vi "Close Reference.vi"(8 "error in (no error)":errorcluster, 11 "Listener In.lvclass":refnum<class "Listener.lvclass">) -> (0 "error out":errorcluster, 3 "Listener out":refnum<class "Listener.lvclass">)   [LabVIEW 2019, in "Listener.lvclass"]
uses:
  Listener.lvclass
  Listener.lvclass/Listener.ctl
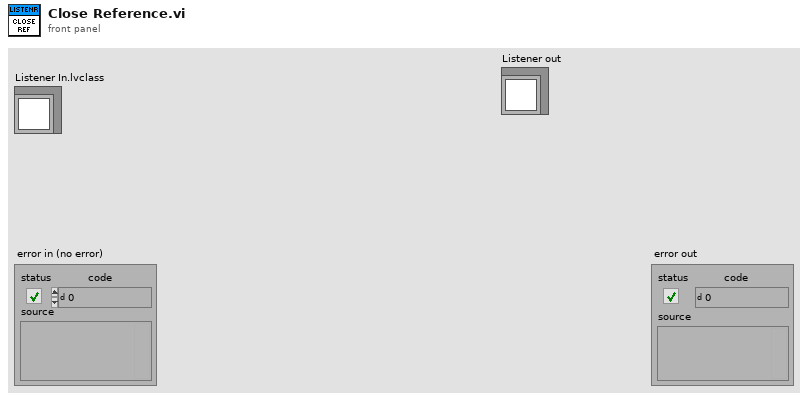
[diagram p1: front panel]
types:
  T1 = typedef "Listener.lvclass/Protocol.ctl" = enum16{"RS-XXX", "AK RS-XXX", "VISA", "TCPIP", "AK TCPIP", "UDP", "GPIB ConvBox"}
  T2 = typedef "Listener.lvclass/TCP Data Structure.ctl" = cluster{"TCP|IP connection ID":refnum<k5>, "IP Address":string, "Port":u16, "Data":string}
  T3 = typedef "Listener.lvclass/UDP Data Structure.ctl" = cluster{"UDP connection ID":refnum<k16>, "Local Address":string, "Local Port":u16, "Target IP Address":string, "Target Port":u16, "Data":string}
  T4 = typedef "Listener.lvclass/AK TCP Data Structure.ctl" = cluster{"TCP|IP connection ID":refnum<k5>, "IP Address":string, "Port":u16, "Data":string, "Current Command Code":string}
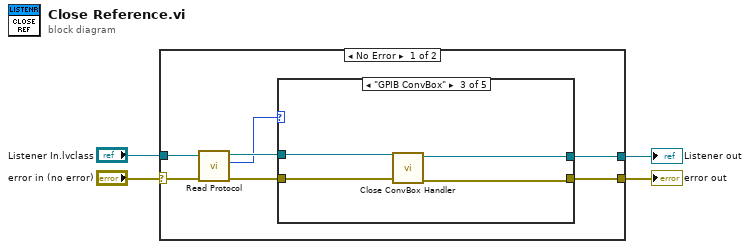
[diagram p0: block diagram]
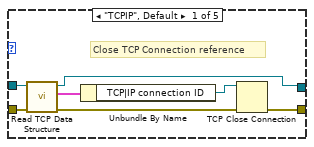
[diagram p2: hidden frame]
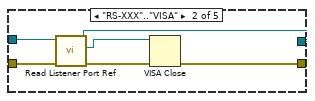
[diagram p3: hidden frame]
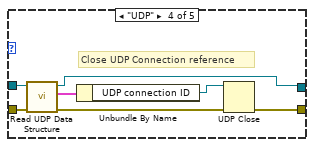
[diagram p4: hidden frame]
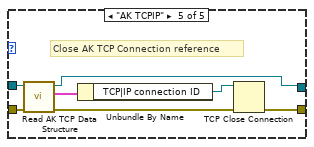
[diagram p5: hidden frame]
diagram:
  n1 = case shown="No Error" "error in (no error)" {
    selector: "error in (no error)" -> [w9 w44]
    tunnel: [w7 w44] -> w3
    tunnel: "Listener In.lvclass" -> [w11 w43]
    tunnel: [w6 w43] -> w1
    frame No Error {
      n2 = call-dynamic "Read Protocol.vi"("error in (no error)"=w9, "Listener in"=w11) -> ("error out"=w8:errorcluster, "Protocol"=w5:T1, "Listener out"=w10:refnum<class "Listener.lvclass">)  [unwired: 7 in]
      n3 = case shown="\"GPIB ConvBox\"" w5 {
        tunnel: w10 -> [w17 w21 w27 w35 w38]
        tunnel: w8 -> [w18 w23 w28 w34 w40]
        tunnel: [w14 w24 w26 w30 w41] -> w7
        tunnel: [w12 w19 w25 w29 w36] -> w6
        frame "TCPIP", Default {
          # "Close TCP Connection reference"
          n4 = call-dynamic "Read TCP Data Structure.vi"("error in (no error)"=w18, "Listener in"=w17) -> ("error out"=w15:errorcluster, "TCP|IP Data Structure"=w16:T2, "Listener out"=w12:refnum<class "Listener.lvclass">)  [unwired: 7 in]
          n5 = Unbundle By Name(w16) -> ("TCP|IP connection ID"=w13:refnum<k5>)
          n6 = TCP Close Connection(connection ID=w13, error in (no error)=w15) -> (error out=w14:errorcluster)  [unwired: 1 in, 1 out]
        }
        frame "RS-XXX".."VISA" {
          n7 = call "Read Listener Port Ref.vi"("error in (no error)"=w23, "Listener in"=w21) -> ("error out"=w22:errorcluster, "Listener Port Ref"=w20:refnum<visa-resource-name>, "Listener out"=w19:refnum<class "Listener.lvclass">)  [unwired: 7 in]
          n8 = VISA Close(VISA resource name=w20, error in (no error)=w22) -> (error out=w24:errorcluster)
        }
        frame "GPIB ConvBox" {
          n9 = call "Close ConvBox Handler.vi"("error in (no error)"=w28, "Listener in"=w27) -> ("error out"=w26:errorcluster, "Listener out"=w25:refnum<class "Listener.lvclass">)  [unwired: 8 in]
        }
        frame "UDP" {
          # "Close UDP Connection reference"
          n10 = call-dynamic "Read UDP Data Structure.vi"("error in (no error)"=w34, "Listener in"=w35) -> ("error out"=w32:errorcluster, "UDP Data Structure"=w33:T3, "Listener out"=w29:refnum<class "Listener.lvclass">)  [unwired: 7 in]
          n11 = Unbundle By Name(w33) -> ("UDP connection ID"=w31:refnum<k16>)
          n12 = UDP Close(connection ID=w31, 8:w32) -> (error out=w30:errorcluster)  [unwired: 1 out]
        }
        frame "AK TCPIP" {
          # "Close AK TCP Connection reference"
          n13 = call-dynamic "Read AK TCP Data Structure.vi"("error in (no error)"=w40, "Listener in"=w38) -> ("error out"=w39:errorcluster, "TCP|IP Data Structure"=w37:T4, "Listener out"=w36:refnum<class "Listener.lvclass">)  [unwired: 7 in]
          n14 = Unbundle By Name(w37) -> ("TCP|IP connection ID"=w42:refnum<k5>)
          n15 = TCP Close Connection(connection ID=w42, error in (no error)=w39) -> (error out=w41:errorcluster)  [unwired: 1 in, 1 out]
        }
      }
    }
    frame Error {
    }
  }
  "error out" <- w3
  "Listener out" <- w1
